vi "test Get Owning Disabled Custom Device.vi"() -> ()   [LabVIEW 2020, in "Scripting.lvclass"]
uses:
  Scripting.lvclass
  Scripting.lvclass/Scripting.ctl
  Scripting/AIM/AIM ARINC 429 Scripting.lvlib
  Shared/VS Channels Definition for Label.ctl
  Shared/Transfer Speed.ctl
  Shared/Direction.ctl
  <vilib>/NI/NI VeriStand Encoding and Decoding/Encoding.ctl
  <vilib>/NI/NI VeriStand Encoding and Decoding/Encoding and Decoding.lvlib
  Shared/Parameter Definition.ctl
  Shared/VS Channel Definition for Parameter.ctl
  Shared/Transfer Type.ctl
  <vilib>/addons/_JKI Toolkits/VI Tester/TestCase.llb/TestCase.lvclass
  C:/Program Files (x86)/National Instruments/LabVIEW 2020/vi.lib/addons/_JKI Toolkits/VI Tester/TestCase.llb/TestCase.lvclass
  C:/dev/git/niveristand-aim-arinc429-custom-device/Source/Custom Device Support/Tests/Unit/Scripting/Scripting.lvclass
panel:
  out "TestCase out":refnum<class "Scripting.lvclass">
  in  "TestCase in":refnum<class "Scripting.lvclass">
  out "error out":errorcluster
  in  "error in":errorcluster
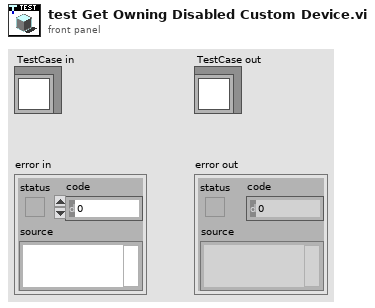
[diagram p1: front panel]
types:
  T1 = typedef "VS Channels Definition for Label.ctl" = cluster{"label (Dec)":u32, "parameters":T2[], "SDI value":u8, "SDI enabled":bool, "transfer type":T5, "create timestamp":bool, "transmit period":u32}
  T2 = typedef "VS Channel Definition for Parameter.ctl" = cluster{"name":string, "unit":string, "Parameter":T3}
  T3 = typedef "Parameter Definition.ctl" = cluster{"start index":i32, "size":i32, "encoding":T4, "signed":bool, "scale multiplier":dbl, "scale offset":dbl, "default value":dbl}
  T4 = typedef "Encoding and Decoding.lvlib/Encoding.ctl" = enum16{"BNR", "BCD", "Discrete"}
  T5 = typedef "Transfer Type.ctl" = enum16{"Scheduled", "Acyclic", "Block", "Strobe"}
  T6 = typedef "Transfer Speed.ctl" = enum16{"LO (12.5 kb/s)", "HI (100 kb/s)"}
  T7 = typedef "Direction.ctl" = enum16{"Rx", "Tx"}
  T8 = typedef "Custom Device API.lvlib/Custom Device Item Ref.ctl" = u64
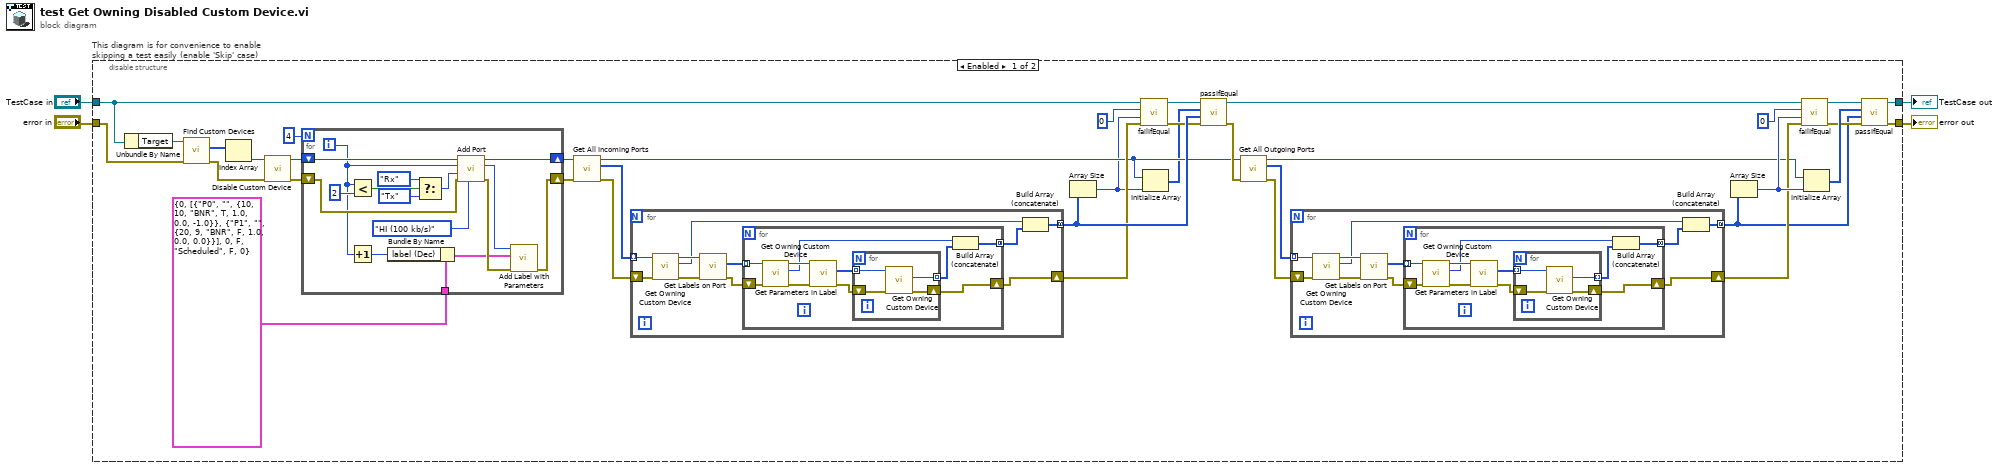
[diagram p0: block diagram]
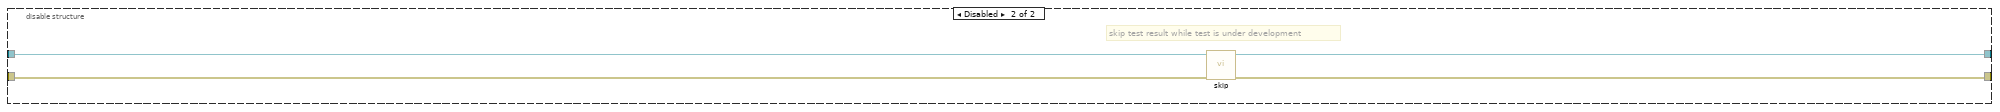
[diagram p2: hidden frame]
diagram:
  n1 = disable-structure "This diagram is for convenience to enable skipping a test easily (enable 'Skip' case)" shown="Enabled" {
    disable-tunnel: "TestCase in" -> [w32 w108]
    disable-tunnel: [w14 w106] -> w1
    disable-tunnel: [w15 w107] -> w3
    disable-tunnel: "error in" -> [w37 w105]
    frame Enabled {
      n2 = Unbundle By Name(w32) -> ("Target"=w40:refnum<k24>)
      n3 = call "Find Custom Devices.vi"("error in"=w37, "target"=w40) -> ("error out"=w8:errorcluster, "AIM ARINC 429 custom devices"=w13:T8[])  [unwired: 7 in, 1 out]
      n4 = Index Array(array=w13) -> (element=w7:T8)  [unwired: 1 in]
      n5 = call "Disable Custom Device.vi"("error in (no error)"=w8, "AIM ARINC 429 ref"=w7) -> ("error out"=w5:errorcluster, "AIM ARINC 429 ref out"=w6:T8)  [unwired: 8 in]
      n6 = for {
        N: 4 -> [_]
        shift-right: [w55] -> w12
        shift-left: w6 -> [w56]
        shift-right: [w42] -> w10
        shift-left: w5 -> [w49]
        tunnel: T1 {"label (Dec)"=0, "parameters"=[{"name"="P0", "unit"="", "Parameter"={"start index"=10, "size"=10, "encoding"=enum."BNR", "signed"=TRUE, "scale multiplier"=1.0, "scale offset"=0.0, "default value"=-1.0}}, {"name"="P1", "unit"="", "Parameter"={"start index"=20, "size"=9, "encoding"=enum."BNR", "signed"=FALSE, "scale multiplier"=1.0, "scale offset"=0.0, "default value"=0.0}}], "SDI value"=0, "SDI enabled"=FALSE, "transfer type"=enum."Scheduled", "create timestamp"=FALSE, "transmit period"=0} ("label") -> [w43]
        i -> [w46]
        n7 = Less?(x=w46, y=2) -> (x < y?=w53:bool)
        n8 = Increment(x=w46) -> (x+1=w45:i32)
        n9 = Bundle By Name(cluster=w43, "label (Dec)"=w45) -> (w44:T1)
        n10 = Select(t=Direction."Rx" ("direction"), s=w53, f=Direction."Tx" ("direction")) -> (s? t:f=w50:T7)
        n11 = call "Add Port.vi"("speed"=Transfer_Speed."HI (100 kb/s)", "error in"=w49, "direction"=w50, "port number"=w46, "custom device ref"=w56) -> ("error out"=w47:errorcluster, "port"=w48:T8, "custom device ref out"=w55:T8)  [unwired: 4 in]
        n12 = call "Add Label with Parameters.vi"("error in"=w47, "label"=w44, "port ref"=w48) -> ("error out"=w42:errorcluster)  [unwired: 7 in, 1 out]
      }
      n13 = call "Get All Incoming Ports.vi"("error in"=w10, "custom device ref"=w12) -> ("error out"=w39:errorcluster, "incoming ports"=w38:T8[], "custom device ref out"=w29:T8)  [unwired: 7 in]
      n14 = for {
        tunnel: w38 -> [w90] mode=indexing
        shift-right: [w84] -> w31
        shift-left: w39 -> [w89]
        tunnel: [w81] -> w35 mode=concatenating
        n15 = call "Get Owning Custom Device.vi"("error in"=w89, "item ref in"=w90) -> ("error out"=w87:errorcluster, "owning AIM ARINC-429 custom device"=w82:T8, "item ref out"=w88:T8)  [unwired: 7 in]
        n16 = call "Get Labels on Port.vi"("error in"=w87, "port ref"=w88) -> ("error out"=w85:errorcluster, "labels"=w86:T8[])  [unwired: 6 in, 2 out]
        n17 = for {
          tunnel: w86 -> [w100] mode=indexing
          shift-right: [w96] -> w84
          shift-left: w85 -> [w98]
          tunnel: [w91] -> w83 mode=concatenating
          n18 = call "Get Owning Custom Device.vi"("error in"=w98, "item ref in"=w100) -> ("error out"=w97:errorcluster, "owning AIM ARINC-429 custom device"=w93:T8, "item ref out"=w99:T8)  [unwired: 7 in]
          n19 = call "Get Parameters in Label.vi"("error in"=w97, "label ref"=w99) -> ("error out"=w94:errorcluster, "parameters"=w95:T8[])  [unwired: 6 in, 2 out]
          n20 = for {
            tunnel: w95 -> [w104] mode=indexing
            tunnel: [w103] -> w92 mode=indexing
            shift-right: [w101] -> w96
            shift-left: w94 -> [w102]
            n21 = call "Get Owning Custom Device.vi"("error in"=w102, "item ref in"=w104) -> ("error out"=w101:errorcluster, "owning AIM ARINC-429 custom device"=w103:T8)  [unwired: 7 in, 1 out]
          }
          n22 = Build Array (concatenate)(w93, w92) -> (w91:T8[])
        }
        n23 = Build Array (concatenate)(w82, w83) -> (w81:T8[])
      }
      n24 = Array Size(array=w35) -> (size(s)=w28:i32)
      n25 = call-dynamic "failIfEqual.vi"("error in (no error)"=w31, "y"=w28, "x"=0 ("size(s)"), "TestCase in"=w32) -> ("error out"=w30:errorcluster, "TestCase out"=w33:refnum<class "Scripting.lvclass">)  [unwired: 6 in]
      n26 = Initialize Array(w29, w28) -> (w27:T8[])
      n27 = call-dynamic "passIfEqual.vi"("error in (no error)"=w30, "y"=w35, "x"=w27, "TestCase in"=w33) -> ("error out"=w36:errorcluster, "TestCase out"=w17:refnum<class "Scripting.lvclass">)  [unwired: 6 in]
      n28 = call "Get All Outgoing Ports.vi"("error in"=w36, "custom device ref"=w29) -> ("error out"=w19:errorcluster, "outgoing ports"=w18:T8[], "custom device ref out"=w16:T8)  [unwired: 7 in]
      n29 = for {
        tunnel: w18 -> [w66] mode=indexing
        shift-right: [w60] -> w23
        shift-left: w19 -> [w65]
        tunnel: [w57] -> w20 mode=concatenating
        n30 = call "Get Owning Custom Device.vi"("error in"=w65, "item ref in"=w66) -> ("error out"=w63:errorcluster, "owning AIM ARINC-429 custom device"=w58:T8, "item ref out"=w64:T8)  [unwired: 7 in]
        n31 = call "Get Labels on Port.vi"("error in"=w63, "port ref"=w64) -> ("error out"=w61:errorcluster, "labels"=w62:T8[])  [unwired: 6 in, 2 out]
        n32 = for {
          tunnel: w62 -> [w76] mode=indexing
          shift-right: [w72] -> w60
          shift-left: w61 -> [w74]
          tunnel: [w67] -> w59 mode=concatenating
          n33 = call "Get Owning Custom Device.vi"("error in"=w74, "item ref in"=w76) -> ("error out"=w73:errorcluster, "owning AIM ARINC-429 custom device"=w69:T8, "item ref out"=w75:T8)  [unwired: 7 in]
          n34 = call "Get Parameters in Label.vi"("error in"=w73, "label ref"=w75) -> ("error out"=w70:errorcluster, "parameters"=w71:T8[])  [unwired: 6 in, 2 out]
          n35 = for {
            tunnel: w71 -> [w80] mode=indexing
            tunnel: [w79] -> w68 mode=indexing
            shift-right: [w77] -> w72
            shift-left: w70 -> [w78]
            n36 = call "Get Owning Custom Device.vi"("error in"=w78, "item ref in"=w80) -> ("error out"=w77:errorcluster, "owning AIM ARINC-429 custom device"=w79:T8)  [unwired: 7 in, 1 out]
          }
          n37 = Build Array (concatenate)(w69, w68) -> (w67:T8[])
        }
        n38 = Build Array (concatenate)(w58, w59) -> (w57:T8[])
      }
      n39 = Array Size(array=w20) -> (size(s)=w25:i32)
      n40 = call-dynamic "failIfEqual.vi"("error in (no error)"=w23, "y"=w25, "x"=0 ("size(s)"), "TestCase in"=w17) -> ("error out"=w24:errorcluster, "TestCase out"=w22:refnum<class "Scripting.lvclass">)  [unwired: 6 in]
      n41 = Initialize Array(w16, w25) -> (w26:T8[])
      n42 = call-dynamic "passIfEqual.vi"("error in (no error)"=w24, "y"=w20, "x"=w26, "TestCase in"=w22) -> ("error out"=w15:errorcluster, "TestCase out"=w14:refnum<class "Scripting.lvclass">)  [unwired: 6 in]
    }
    frame Disabled {
      # "skip test result while test is under development"
      n43 = call <vilib>:"skip.vi"("error in (no error)"=w105, "TestCase in"=w108) -> ("error out"=w107:errorcluster, "TestCase out"=w106:refnum<class "Scripting.lvclass">)  [unwired: 8 in]
    }
  }
  "error out" <- w3
  "TestCase out" <- w1
